vi "Log FA Data.vi"() -> ()   [LabVIEW 2011]
panel:
  out "Waveform Graph":i32[](graph)
  in  "BPM and PS Data":dbl[][](array[numeric])
  out "Writting file?":bool
  in  "Start":bool caption="START"
  in  "Maximum number of files":i32=5760
  in  "Number of measurements":i32=100000
  in  "FOFB Controller IP":string="10.0.18.132"
  in  "Data path":string="C:\\Data\\"
  in  "stop":bool
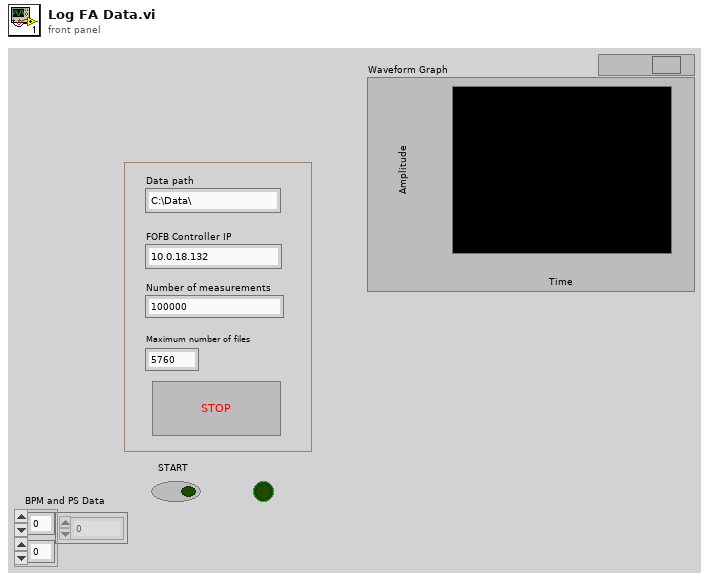
[diagram p1: front panel]
types:
  T1 = enum16{"Idle", "Wait Connection", "Read Data", "Close Connection"}
  T2 = typedef "Type HDF IDs.ctl" = cluster{"File":i32, "BPM":i32, "BPM Horizontal":i32, "BPM Vertical":i32, "Correctors":i32, "Correctors Setpoint":i32, "Correctors Setpoint ACH":i32, "Correctors Setpoint ACV":i32, "Correctors Setpoint ALV":i32, "Correctors Reading":i32, "Correctors Reading ACH":i32, "Correctors Reading ACV":i32, "Correctors Reading ALV":i32, "Dataset IDs":i32[], "Plist":i32[], "Space IDs":i32[]}
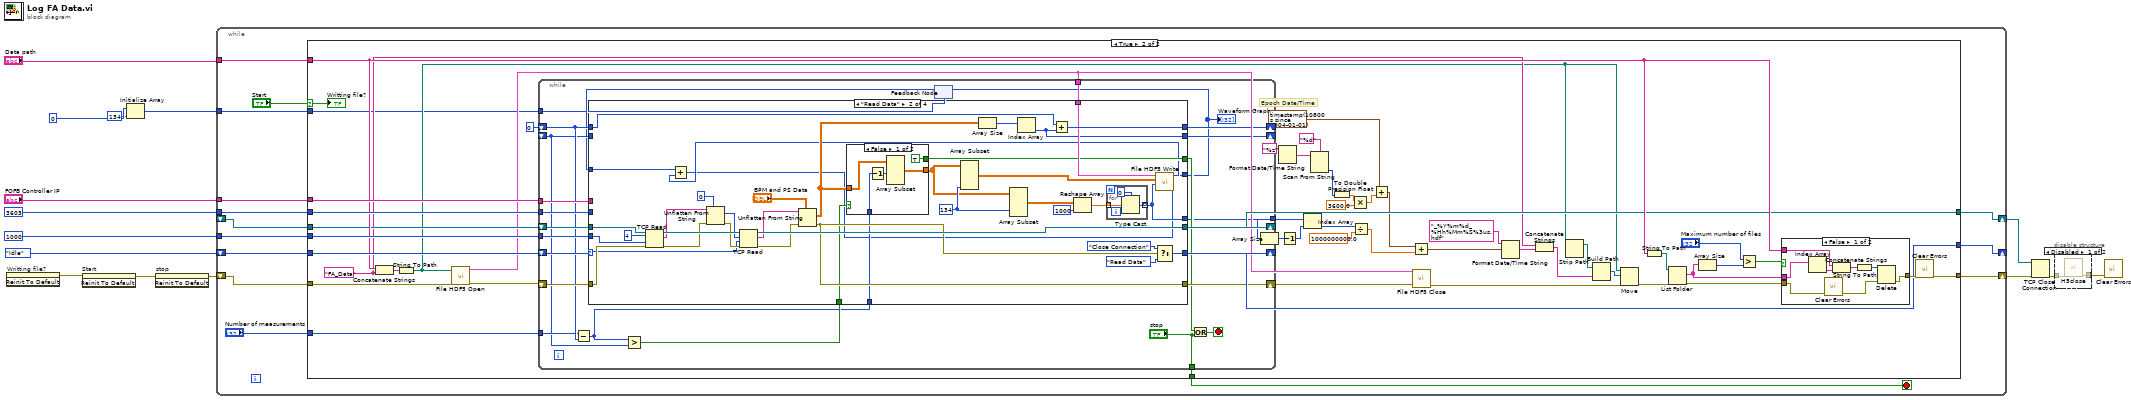
[diagram p0: block diagram]
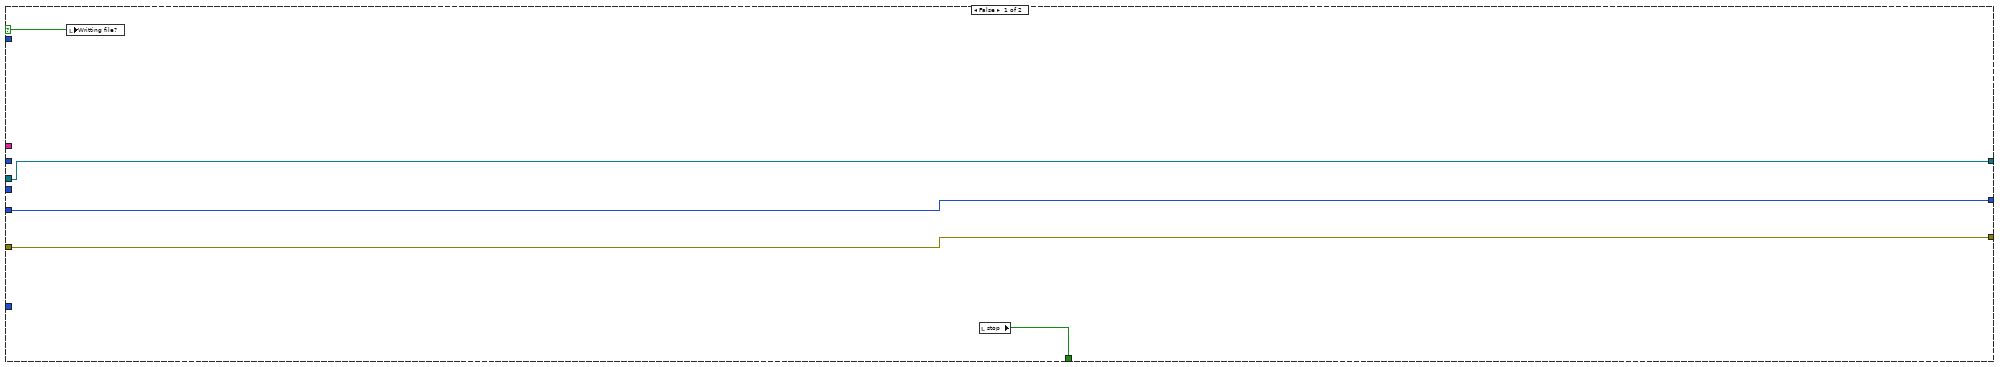
[diagram p3: hidden frame]
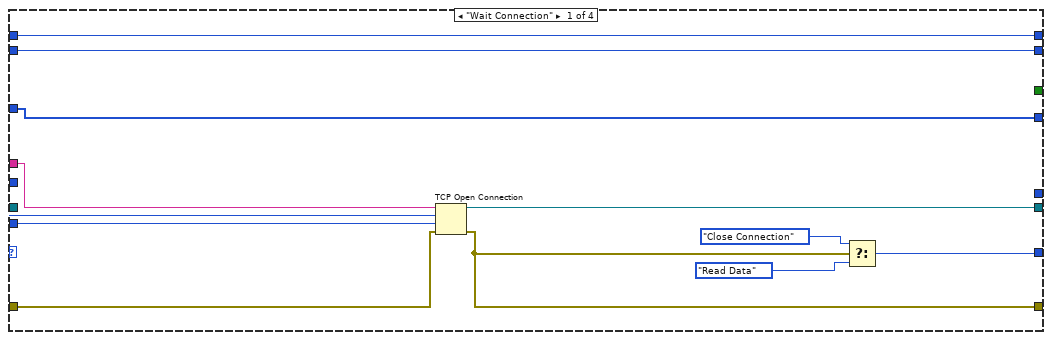
[diagram p5: hidden frame]
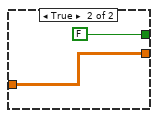
[diagram p6: hidden frame]
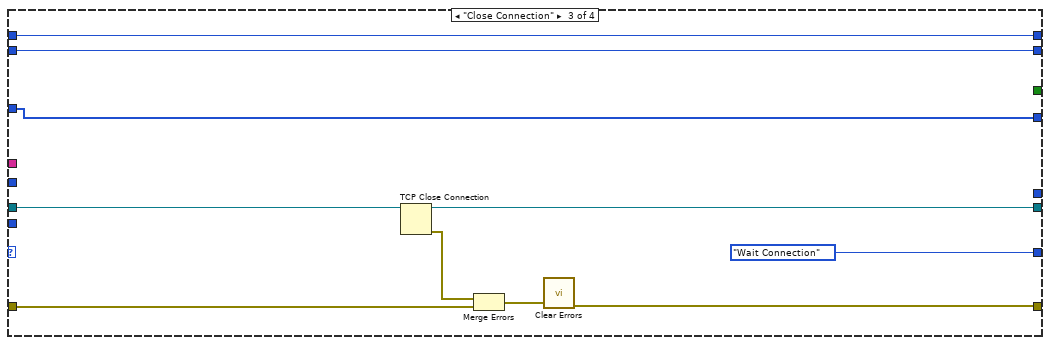
[diagram p7: hidden frame]
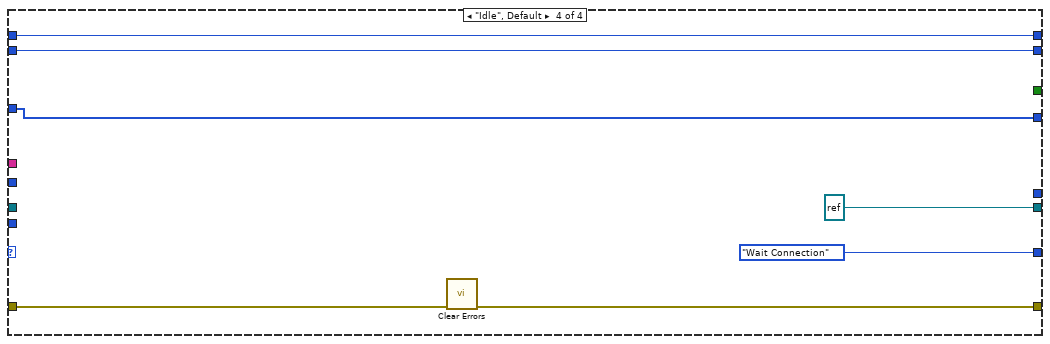
[diagram p8: hidden frame]
diagram:
  n1 = invoke on="Writting file?" class="Bool (strict)" method="Reinit To Default"() -> (error out=w10:errorcluster)  [unwired: 3 in, 2 out]
  n2 = invoke on="Start" class="Bool (strict)" method="Reinit To Default"(error in=w10) -> (error out=w4:errorcluster)  [unwired: 2 in, 2 out]
  n3 = Initialize Array(0, 134 ("dimension size")) -> (w1:i32[])
  n4 = invoke on="stop" class="Bool (strict)" method="Reinit To Default"(error in=w4) -> (error out=w5:errorcluster)  [unwired: 2 in, 2 out]
  n5 = while {
    tunnel: "FOFB Controller IP" -> [w29]
    tunnel: u16 3603 ("TCP Port") -> [w28]
    tunnel: 1000 ("TCP Listening Timeout") -> [w27]
    tunnel: "Data path" -> [w25]
    shift-right: [w23] -> w6
    shift-left: w5 -> [w20]
    shift-right: [w24] -> w7
    shift-left: _ -> [w19]
    shift-right: [w18] -> _
    shift-left: T1."Idle" ("f") -> [w26]
    tunnel: w1 -> [w16]
    stop <- w21 stop-if-true
    n6 = case shown="True" "Start" {
      selector: "Start" -> [w34 w62]
      tunnel: w29 -> [_ w85]
      tunnel: w28 -> [_ w84]
      tunnel: w27 -> [_ w83]
      tunnel: w26 -> [w31 w82]
      tunnel: w25 -> [_ w70]
      tunnel: w20 -> [w32 w52]
      tunnel: "Number of measurements" -> [_ w67]
      tunnel: [w30 w65] -> w24
      tunnel: [w32 w63] -> w23
      tunnel: [w33 w61] -> w21
      tunnel: w19 -> [w30 w60]
      tunnel: [w31 w59] -> w18
      tunnel: w16 -> [_ w35]
      frame False {
        n7 = local write "Writting file?"(w34) -> ()
        n8 = local read "stop"() -> (w33:bool)
      }
      frame True {
        w58 = "FA_Data" ("FOFB Controller IP")
        # "Epoch Date/Time"
        n9 = Concatenate Strings(w70, w58) -> (w81:string)
        n10 = String To Path(string=w81) -> (path=w57:path)
        n11 = call "File HDF5 Open.vi"("error in (no error)"=w52, "File Path"=w57) -> ("error out"=w56:errorcluster, "HDF IDs out"=w53:T2)  [unwired: 8 in]
        n12 = while {
          shift-right: [w110] -> w55
          shift-left: w56 -> [w118]
          shift-right: [w114] -> w59
          shift-left: w82 -> [w116]
          shift-right: [w115] -> w65
          shift-left: w60 -> [w117]
          tunnel: w85 -> [w113]
          tunnel: w84 -> [w112]
          tunnel: w83 -> [w111]
          shift-right: [w109] -> _
          shift-left: 0 -> [w103]
          tunnel: w67 -> [w102]
          tunnel: ["stop"] -> w61
          tunnel: w53 -> [w106]
          shift-right: [w105] -> _
          shift-left: _ -> [w100]
          tunnel: [w98] -> w40
          tunnel: w35 -> [w96]
          stop <- w108 stop-if-true
          n13 = Subtract(x=w102, y=w103) -> (x-y=w101:i32)
          n14 = Greater?(x=w101, y=w100) -> (0:w104:bool)
          n15 = feedback #1(w96) -> (w97:i32[])
          n16 = case shown="\"Read Data\"" w116 {
            tunnel: [w130 w167 w187 refnum<k5> refnum ("connection ID")] -> w115
            tunnel: [w129 w166 T1."Wait Connection" ("f") T1."Wait Connection" ("f")] -> w114
            tunnel: [w123 w152 w181 w191] -> w110
            tunnel: w118 -> [w128 w163 w183 w192]
            tunnel: w117 -> [_ w164 w186 _]
            tunnel: w113 -> [w125 _ _ _]
            tunnel: w112 -> [w124 _ _ _]
            tunnel: w111 -> [w122 w151 _ _]
            tunnel: [w121 w150 w180 w190] -> w109
            tunnel: w103 -> [w121 w149 w180 w190]
            tunnel: w106 -> [_ w148 _ _]
            tunnel: [w120 w146 w179 w189] -> w105
            tunnel: w104 -> [_ w145 _ _]
            tunnel: w101 -> [_ w144 _ _]
            tunnel: w100 -> [w120 _ w179 w189]
            tunnel: [_ w143 _ _] -> w99
            tunnel: [_ w135 _ _] -> w98
            tunnel: [w119 w131 w178 w188] -> w95
            tunnel: w97 -> [w119 w132 w178 w188]
            frame "Wait Connection" {
              n17 = TCP Open Connection(address=w125, remote port or service name=w124, timeout ms (60000)=w122, error in (no error)=w128) -> (connection ID=w130:refnum<k5>, error out=w123:errorcluster)  [unwired: 1 in]
              n18 = Select(t=T1."Close Connection" ("f"), s=w123, f=T1."Read Data") -> (s? t:f=w129:T1)
            }
            frame "Read Data" {
              w140 = 134 ("index (row)")
              n19 = TCP Read(connection ID=w164, bytes to read=4, error in (no error)=w163, 9:w151) -> (connection ID out=w165:refnum<k5>, data out=w159:string, error out=w153:errorcluster)  [unwired: 1 in]
              n20 = Unflatten From String(type=0 ("bytes to read"), binary string=w159, error in (no error)=w153) -> (value=w157:i32, error out=w155:errorcluster)  [unwired: 2 in, 1 out]
              n21 = TCP Read(connection ID=w165, bytes to read=w157, error in (no error)=w155, 9:w151) -> (connection ID out=w167:refnum<k5>, data out=w156:string, error out=w154:errorcluster)  [unwired: 1 in]
              n22 = Unflatten From String(type="BPM and PS Data", binary string=w156, error in (no error)=w154) -> (value=w141:dbl[][], error out=w152:errorcluster)  [unwired: 2 in, 1 out]
              n23 = case shown="False" w145 {
                tunnel: w141 -> [w175 w177]
                tunnel: [w174 w177] -> w138
                tunnel: w144 -> [w172 _]
                tunnel: [TRUE ("x") FALSE ("x")] -> w143
                frame False {
                  n24 = Decrement(x=w172) -> (x-1=w171:i32)
                  n25 = Array Subset(array=w175, length (row)=w171) -> (w174:dbl[][])  [unwired: 3 in]
                }
                frame True {
                }
              }
              n26 = Array Subset(array=w138, length (col)=w140) -> (w137:dbl[][])  [unwired: 3 in]
              n27 = Array Size(array=w141) -> (size(s)=w147:i32[])
              n28 = Array Subset(array=w138, index (col)=w140) -> (w139:dbl[][])  [unwired: 3 in]
              n29 = Index Array(array=w147) -> (element=w146:i32)  [unwired: 1 in]
              n30 = Add(x=w149, y=w146) -> (x+y=w150:i32)
              n31 = Reshape Array(w139, 1000 ("dimension size")) -> (w134:dbl[])
              n32 = for {
                tunnel: [w169] -> w135 mode=indexing
                tunnel: w134 -> [w168] mode=indexing
                n33 = Type Cast(type=u64 0 ("unsigned 64bit integer"), x=w168) -> (*(type *) &x=w169:u64)
              }
              n34 = call "File HDF5 Write.vi"("Timestamp"=w135, "BPM and PS Data"=w137, "HDF IDs in"=w148) -> ("Array"=w133:i32[])  [unwired: 8 in]
              n35 = Add(x=w132, y=w133) -> (x+y=w131:i32[])
              n36 = Select(t=T1."Close Connection" ("f"), s=w152, f=T1."Read Data") -> (s? t:f=w166:T1)
            }
            frame "Close Connection" {
              n37 = TCP Close Connection(connection ID=w186) -> (connection ID out=w187:refnum<k5>, error out=w184:errorcluster)  [unwired: 2 in]
              n38 = Merge Errors(w184, w183) -> (w182:errorcluster)
              n39 = call <vilib>:"Clear Errors.vi"("error in (no error)"=w182) -> ("error out"=w181:errorcluster)  [unwired: 6 in]
            }
            frame "Idle", Default {
              n40 = call <vilib>:"Clear Errors.vi"("error in (no error)"=w192) -> ("error out"=w191:errorcluster)  [unwired: 6 in]
            }
          }
          "Waveform Graph" <- w95
          n41 = feedback-in #1(w95) -> ()
          n42 = Or(x=w99, y="stop") -> (x .or. y?=w108:bool)
        }
        n43 = Array Size(array=w40) -> (size(s)=w39:i32)
        n44 = Format Date/Time String(time format string (%c)="%z") -> (date/time string=w49:string)  [unwired: 2 in]
        n45 = Decrement(x=w39) -> (x-1=w38:i32)
        n46 = Index Array(array=w40, index=w38) -> (element=w36:u64)
        n47 = Scan From String(format string="%d", input string=w49) -> (output 1=w47:i32)  [unwired: 3 in, 3 out]
        n48 = To Double Precision Float(number=w47) -> (double precision float=w42:dbl)
        n49 = Multiply(x=w42, y=3600.0) -> (x*y=w43:dbl)
        n50 = Divide(x=w36, y=1000000000.0) -> (x/y=w37:dbl)
        n51 = Add(x=timestamp(10800 s since 1904-01-01) ("time stamp"), y=w43) -> (x+y=w44:timestamp)
        n52 = Add(x=w44, y=w37) -> (x+y=w46:timestamp)
        n53 = call "File HDF5 Close.vi"("error in (no error)"=w55, "HDF IDs in"=w53) -> ("error out"=w54:errorcluster)  [unwired: 9 in]
        n54 = Format Date/Time String(time format string (%c)="_%Y%m%d_%Hh%Mm%S%3us.hdf", seconds (now)=w46) -> (date/time string=w78:string)  [unwired: 1 in]
        n55 = Concatenate Strings(w58, w78) -> (w76:string)
        n56 = Strip Path(path=w57) -> (stripped path=w68:path)  [unwired: 1 out]
        n57 = Build Path(base path=w68, name or relative path=w76) -> (appended path=w79:path)
        n58 = Move(source path=w57, error in=w54, 10:w79) -> (error out=w69:errorcluster)  [unwired: 2 in, 2 out]
        n59 = String To Path(string=w70) -> (path=w71:path)
        n60 = List Folder(path=w71, error in=w69) -> (filenames=w72:string[], error out=w66:errorcluster)  [unwired: 2 in, 2 out]
        n61 = Array Size(array=w72) -> (size(s)=w74:i32)
        n62 = Greater?(x="Maximum number of files", y=w74) -> (0:w73:bool)
        n63 = case shown="False" w73 {
          tunnel: w72 -> [w93 _]
          tunnel: w70 -> [w91 _]
          tunnel: w66 -> [w87 w94]
          tunnel: [w88 w94] -> w64
          frame False {
            n64 = Index Array(array=w93) -> (element=w92:string)  [unwired: 1 in]
            n65 = call <vilib>:"Clear Errors.vi"("error in (no error)"=w87) -> ("error out"=w86:errorcluster)  [unwired: 6 in]
            n66 = Concatenate Strings(w91, w92) -> (w89:string)
            n67 = String To Path(string=w89) -> (path=w90:path)
            n68 = Delete(path (use dialog)=w90, error in=w86) -> (error out=w88:errorcluster)  [unwired: 3 in, 2 out]
          }
          frame True {
          }
        }
        n69 = call <vilib>:"Clear Errors.vi"("error in (no error)"=w64) -> ("error out"=w63:errorcluster)  [unwired: 6 in]
        "Writting file?" <- w62
      }
    }
  }
  n70 = TCP Close Connection(connection ID=w7, error in (no error)=w6) -> (error out=w9:errorcluster)  [unwired: 1 in, 1 out]
  n71 = disable-structure shown="Disabled" {
    disable-tunnel: w9 -> [w196 w197]
    disable-tunnel: [w195 w197] -> w8
    frame Disabled {
      n72 = call <instrlib>:"H5close.vi"("error in (no error)"=w196) -> ("error out"=w195:errorcluster)  [unwired: 10 in]
    }
    frame Enabled {
    }
  }
  n73 = call <vilib>:"Clear Errors.vi"("error in (no error)"=w8) -> ()  [unwired: 6 in, 1 out]
